vi "ubinary_save.vi"(8 "error in":errorcluster, 10 "file (use dialog)":path, 11 "VI":refnum<vi>) -> (0 "error out":errorcluster)   [LabVIEW 2012]
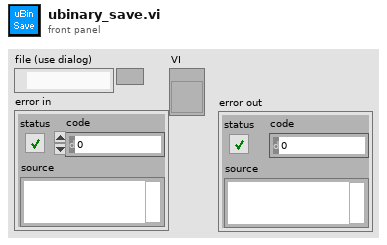
[diagram p1: front panel]
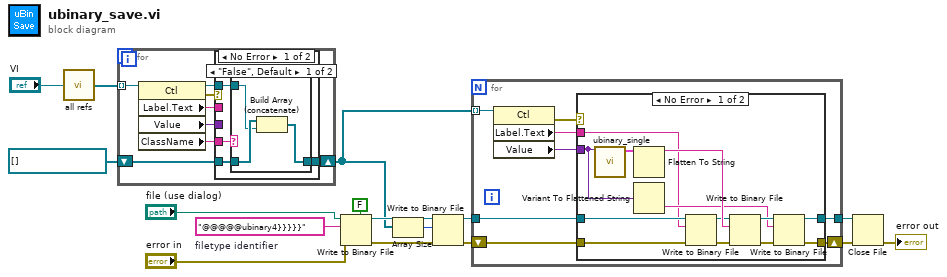
[diagram p0: block diagram]
diagram:
  w10 = "@@@@@ubinary4}}}}}"  # filetype identifier
  n1 = call "all refs.vi"("VI"="VI") -> ("all controls"=w2:refnum<vi>[])
  n2 = for {
    tunnel: w2 -> [w23] mode=indexing
    shift-right: [w19] -> w4
    shift-left: refnum<vi>[] [] ("ControlsOnPage") -> [w18]
    n3 = property class="Ctl"(reference=w23) -> (reference out=w17:refnum<vi>, error out=w24:errorcluster, "Label.Text"=w21:string, "Value"=w22:variant, "ClassName"=w20:string)  [unwired: 1 in]
    n4 = case shown="No Error" w24 {
      tunnel: w22 -> [_ _]
      tunnel: w21 -> [_ _]
      tunnel: w20 -> [w28 _]
      tunnel: [w26 w33] -> w19
      tunnel: w18 -> [w27 w33]
      tunnel: w17 -> [w25 _]
      frame No Error {
        n5 = case shown="\"False\", Default" w28 {
          tunnel: w27 -> [w31 w32]
          tunnel: [w29 w32] -> w26
          tunnel: w25 -> [w30 _]
          frame "False", Default {
            n6 = Build Array (concatenate)(w31, w30) -> (w29:refnum<vi>[])
          }
          frame "" {
          }
        }
      }
      frame Error {
      }
    }
  }
  n7 = Write to Binary File(file (use dialog)="file (use dialog)", data=w10, error in="error in", 5:FALSE ("prepend array or string size? (T)")) -> (refnum out=w11:refnum<file>, error out=w9:errorcluster)  [unwired: 2 in, 1 out]
  n8 = Array Size(array=w4) -> (size(s)=w3:i32)
  n9 = Write to Binary File(file (use dialog)=w11, data=w3, error in=w9) -> (refnum out=w13:refnum<file>, error out=w14:errorcluster)  [unwired: 3 in, 1 out]
  n10 = for {
    shift-right: [w40] -> w16
    shift-left: w14 -> [w37]
    tunnel: w13 -> [w38]
    tunnel: [w39] -> w15
    tunnel: w4 -> [w35] mode=indexing
    n11 = property class="Ctl"(reference=w35) -> (error out=w34:errorcluster, "Label.Text"=w36:string, "Value"=w41:variant)  [unwired: 1 in, 1 out]
    n12 = case shown="No Error" w34 {
      tunnel: w41 -> [w54 _]
      tunnel: [w50 w55] -> w40
      tunnel: [w48 w56] -> w39
      tunnel: w38 -> [w44 w56]
      tunnel: w37 -> [w43 w55]
      tunnel: w36 -> [w42 _]
      frame No Error {
        n13 = call "ubinary_single.vi"("Cluster"=w54) -> ("Header"=w53:cluster{"Element Names":string[], u8[]})  [unwired: 9 in, 1 out]
        n14 = Flatten To String(anything=w53) -> (data string=w52:string)  [unwired: 3 in, 2 out]
        n15 = Variant To Flattened String(Variant=w54) -> (data string=w47:string)  [unwired: 1 out]
        n16 = Write to Binary File(file (use dialog)=w44, data=w42, error in=w43) -> (refnum out=w45:refnum<file>, error out=w46:errorcluster)  [unwired: 3 in, 1 out]
        n17 = Write to Binary File(file (use dialog)=w45, data=w52, error in=w46) -> (refnum out=w49:refnum<file>, error out=w51:errorcluster)  [unwired: 3 in, 1 out]
        n18 = Write to Binary File(file (use dialog)=w49, data=w47, error in=w51) -> (refnum out=w48:refnum<file>, error out=w50:errorcluster)  [unwired: 3 in, 1 out]
      }
      frame Error {
      }
    }
  }
  n19 = Close File(refnum=w15, error in=w16) -> (error out=→"error out":errorcluster)  [unwired: 1 out]
